vi "Sample Transfer Set Freezer.vi"(7 "Container":T1, 8 "error in (no error)":errorcluster, 10 "ON/OFF(OFF)":bool, 11 "cRIO-CO2 in":refnum<class "cRIO-CO2.lvclass">) -> (0 "error out":errorcluster, 2 "Container Name String":string, 3 "cRIO-CO2 out":refnum<class "cRIO-CO2.lvclass">)   [LabVIEW 2015, in "cRIO-Carbondioxide.lvlib" / "cRIO-CO2.lvlib" / "cRIO-CO2.lvclass"]
uses:
  cRIO-CO2.lvclass
  Controls/Sample Transfer Container Enumerator.ctl
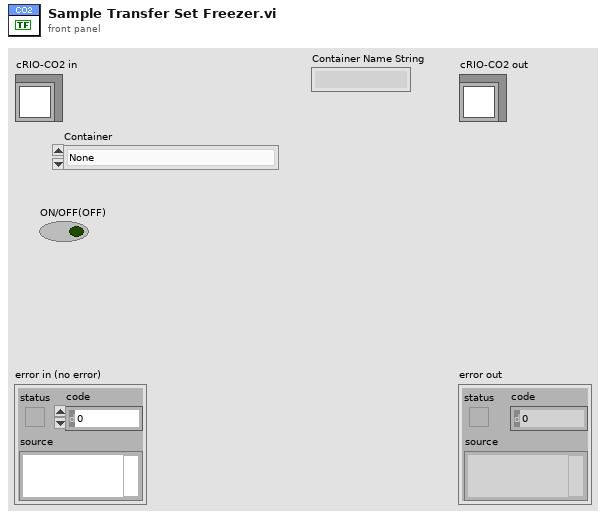
[diagram p1: front panel]
types:
  T1 = typedef "Sample Transfer Container Enumerator.ctl" = enum16{"None", "Sample 1", "Sample 2", "Sample 3", "Sample 4", "Sample 5", "Storage 01", "Storage 02", "Storage 03", "Storage 04", "Storage 05", "Storage 06", "Storage 07", "Storage 08", "Storage 09", "Storage 10", "Storage 11", "Storage 12", "Syringe", "Undefined"}
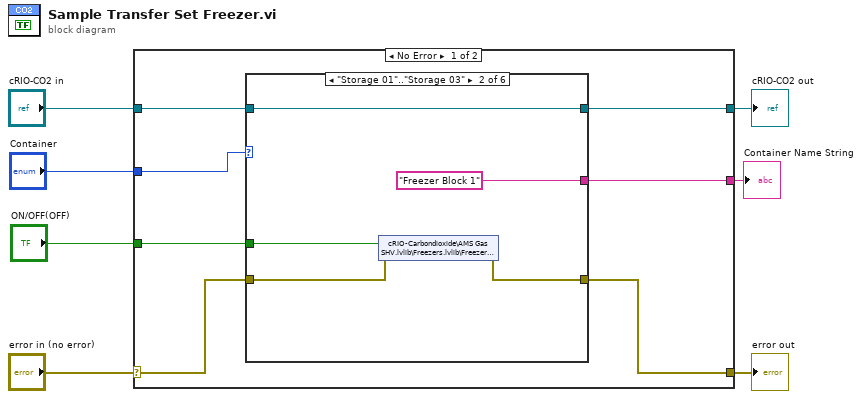
[diagram p0: block diagram]
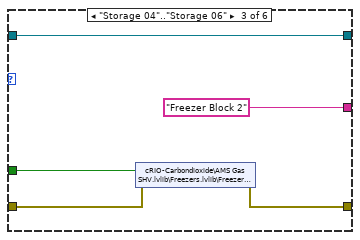
[diagram p3: hidden frame]
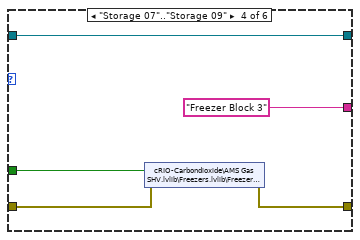
[diagram p4: hidden frame]
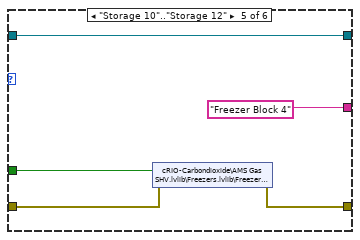
[diagram p5: hidden frame]
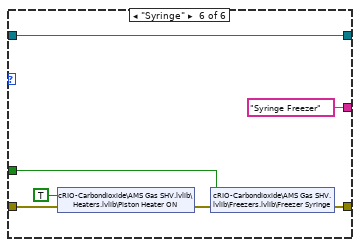
[diagram p6: hidden frame]
diagram:
  n1 = case shown="No Error" "error in (no error)" {
    selector: "error in (no error)" -> [w8 w45]
    tunnel: [w13 w45] -> w6
    tunnel: [w14 w44] -> w4
    tunnel: "cRIO-CO2 in" -> [w12 w44]
    tunnel: "Container" -> [w11 _]
    tunnel: "ON/OFF(OFF)" -> [w10 _]
    tunnel: [w9 _] -> w1
    frame No Error {
      n2 = case shown="\"Storage 01\"..\"Storage 03\"" w11 {
        tunnel: w8 -> [w16 w20 w25 w30 w35 w39]
        tunnel: w12 -> [w15 w21 w26 w31 w36 w43]
        tunnel: [w16 w19 w24 w29 w34 w42] -> w13
        tunnel: [w15 w21 w26 w31 w36 w43] -> w14
        tunnel: w10 -> [_ w18 w23 w28 w33 w40]
        tunnel: [_ "Freezer Block 1" ("string") "Freezer Block 2" ("string") "Freezer Block 3" ("string") "Freezer Block 4" ("string") "Syringe Freezer" ("string")] -> w9
        frame "None", Default {
        }
        frame "Storage 01".."Storage 03" {
          n3 = shared-variable "cRIO-Carbondioxide\\AMS Gas SHV.lvlib\\Freezers.lvlib\\Freezer Tank 1"(w18, error in=w20) -> (error out=w19:errorcluster)
        }
        frame "Storage 04".."Storage 06" {
          n4 = shared-variable "cRIO-Carbondioxide\\AMS Gas SHV.lvlib\\Freezers.lvlib\\Freezer Tank 2"(w23, error in=w25) -> (error out=w24:errorcluster)
        }
        frame "Storage 07".."Storage 09" {
          n5 = shared-variable "cRIO-Carbondioxide\\AMS Gas SHV.lvlib\\Freezers.lvlib\\Freezer Tank 3"(w28, error in=w30) -> (error out=w29:errorcluster)
        }
        frame "Storage 10".."Storage 12" {
          n6 = shared-variable "cRIO-Carbondioxide\\AMS Gas SHV.lvlib\\Freezers.lvlib\\Freezer Tank 4"(w33, error in=w35) -> (error out=w34:errorcluster)
        }
        frame "Syringe" {
          n7 = shared-variable "cRIO-Carbondioxide\\AMS Gas SHV.lvlib\\Heaters.lvlib\\Piston Heater ON"(TRUE ("Piston Heater ON"), error in=w39) -> (error out=w38:errorcluster)
          n8 = shared-variable "cRIO-Carbondioxide\\AMS Gas SHV.lvlib\\Freezers.lvlib\\Freezer Syringe"(w40, error in=w38) -> (error out=w42:errorcluster)
        }
      }
    }
    frame Error {
    }
  }
  "error out" <- w6
  "cRIO-CO2 out" <- w4
  "Container Name String" <- w1
